vi "segmentador de capas.vi"() -> ()   [LabVIEW 2016]
panel:
  in  "Horizontal Pointer Slide":dbl(slide) scale=0.0..255.0
  out "new picture 2":picture
  out "new picture":picture
  in  "File Path Control":path
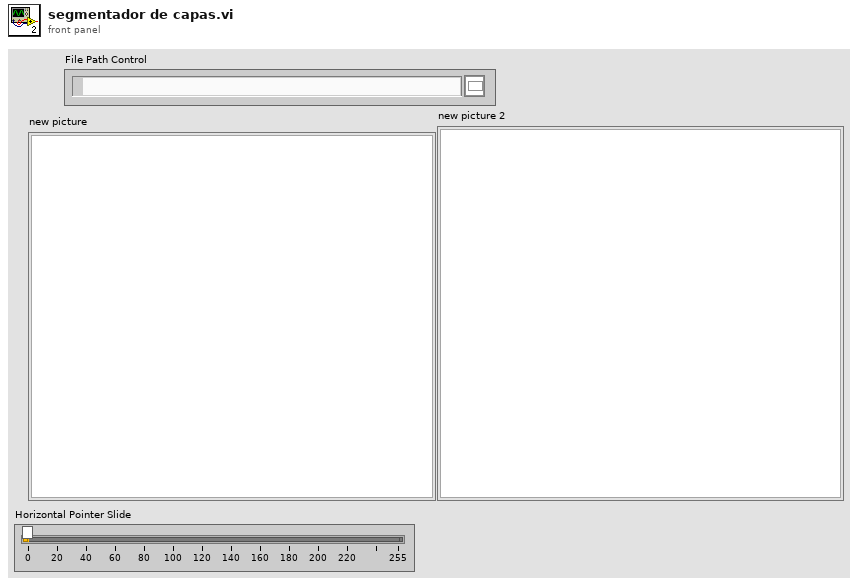
[diagram p1: front panel]
types:
  T1 = typedef "imagedata.ctl" = cluster{"image type":i32, "image depth":i32, "image":u8[], "mask":u8[], "colors":u32[], "Rectangle":cluster{"left":i16, "top":i16, "right":i16, "bottom":i16}}
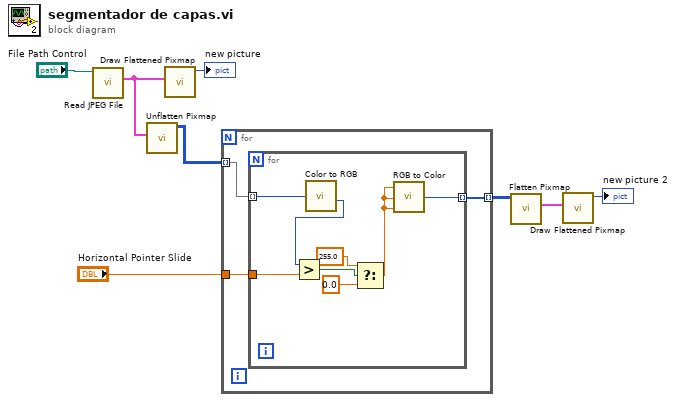
[diagram p0: block diagram]
diagram:
  n1 = call <vilib>:"Read JPEG File.vi"("path to JPEG file"="File Path Control") -> ("image data"=w6:T1)  [unwired: 8 in, 2 out]
  n2 = call <vilib>:"Unflatten Pixmap.vi"("image data"=w6) -> ("24-bit pixmap"=w5:u32[][])  [unwired: 4 in, 6 out]
  n3 = call <vilib>:"Draw Flattened Pixmap.vi"("image data"=w6) -> ("new picture"=→"new picture":picture)  [unwired: 8 in]
  n4 = for {
    tunnel: w5 -> [w11] mode=indexing
    tunnel: [w10] -> w4 mode=indexing
    tunnel: "Horizontal Pointer Slide" -> [w9]
    n5 = for {
      tunnel: w11 -> [w19] mode=indexing
      tunnel: [w18] -> w10 mode=indexing
      tunnel: w9 -> [w13]
      n6 = call <vilib>:"Color to RGB.vi"("Color"=w19) -> ("G"=w12:u8)  [unwired: 3 out]
      n7 = Greater?(x=w12, y=w13) -> (0:w17:bool)
      n8 = Select(t=255.0, s=w17, f=0.0) -> (s? t:f=w14:dbl)
      n9 = call <vilib>:"RGB to Color.vi"("B"=w14, "G"=w14, "R"=w14) -> ("Color"=w18:u32)
    }
  }
  n10 = call <vilib>:"Flatten Pixmap.vi"("24-bit pixmap"=w4) -> ("image data"=w3:T1)  [unwired: 10 in]
  n11 = call <vilib>:"Draw Flattened Pixmap.vi"("image data"=w3) -> ("new picture"=→"new picture 2":picture)  [unwired: 8 in]
